vi "gyro -- async sweeper.vi"(11 "sweeper event pair":T4) -> ()   [LabVIEW 2018]
uses:
  publisher action.ctl
  data source action.ctl
  server talkback message type.ctl
  gyro -- async sweeper parameters.ctl
  freq scan type.ctl
  show-win- control.ctl
  server talkto message type.ctl
  server talk-to-back pair.ctl
panel:
  in  "Tab Control":enum32{"Page 1", "Page 2"}(tab)
  in  "sweeper parameters":T1={"delay-circle(msec)"=0, "N"=300, "scan type"=enum."linear", "gamma factor"=1.5, "history length"=1}
  in  "win":T3={"cen (Hz)"=32757.83435625395, "win (Hz)"=134.34356253945762, "left (Hz)"=32690.66257498422, "right (Hz)"=32825.00613752368}
  out "progress":i32(slide) min=0 max=300 step=1 scale=0.0..300.0
  out "stopped?":bool=TRUE
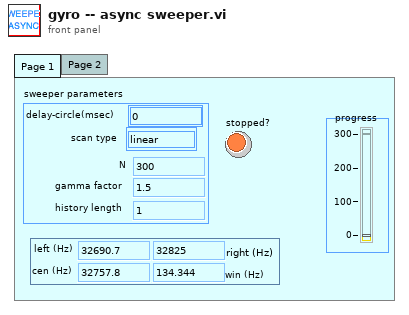
[diagram p1: front panel]
types:
  T1 = typedef "gyro -- async sweeper parameters.ctl" = cluster{"delay-circle(msec)":i64, "N":i64, "scan type":T2, "gamma factor":dbl, "history length":i64}
  T2 = typedef "freq scan type.ctl" = enum16{"linear", "arctan"}
  T3 = typedef "show-win- control.ctl" = cluster{"cen (Hz)":dbl, "win (Hz)":dbl, "left (Hz)":dbl, "right (Hz)":dbl}
  T4 = typedef "server talk-to-back pair.ctl" = cluster{"talkback event":refnum<user-event>, "talkto event":refnum<user-event>}
  T5 = typedef "publisher action.ctl" = enum16{"set", "get", "init", "check"}
  T6 = typedef "server talkback message type.ctl" = cluster{"message":enum16{"new", "void"}}
  T7 = typedef "data source action.ctl" = enum16{"set", "get", "init", "set-and-get", "init source"}
  T8 = enum16{"stop", "start", "update pars", "update request", "new", "launch", "exit", "get", "reset", "pause", "unpause"}
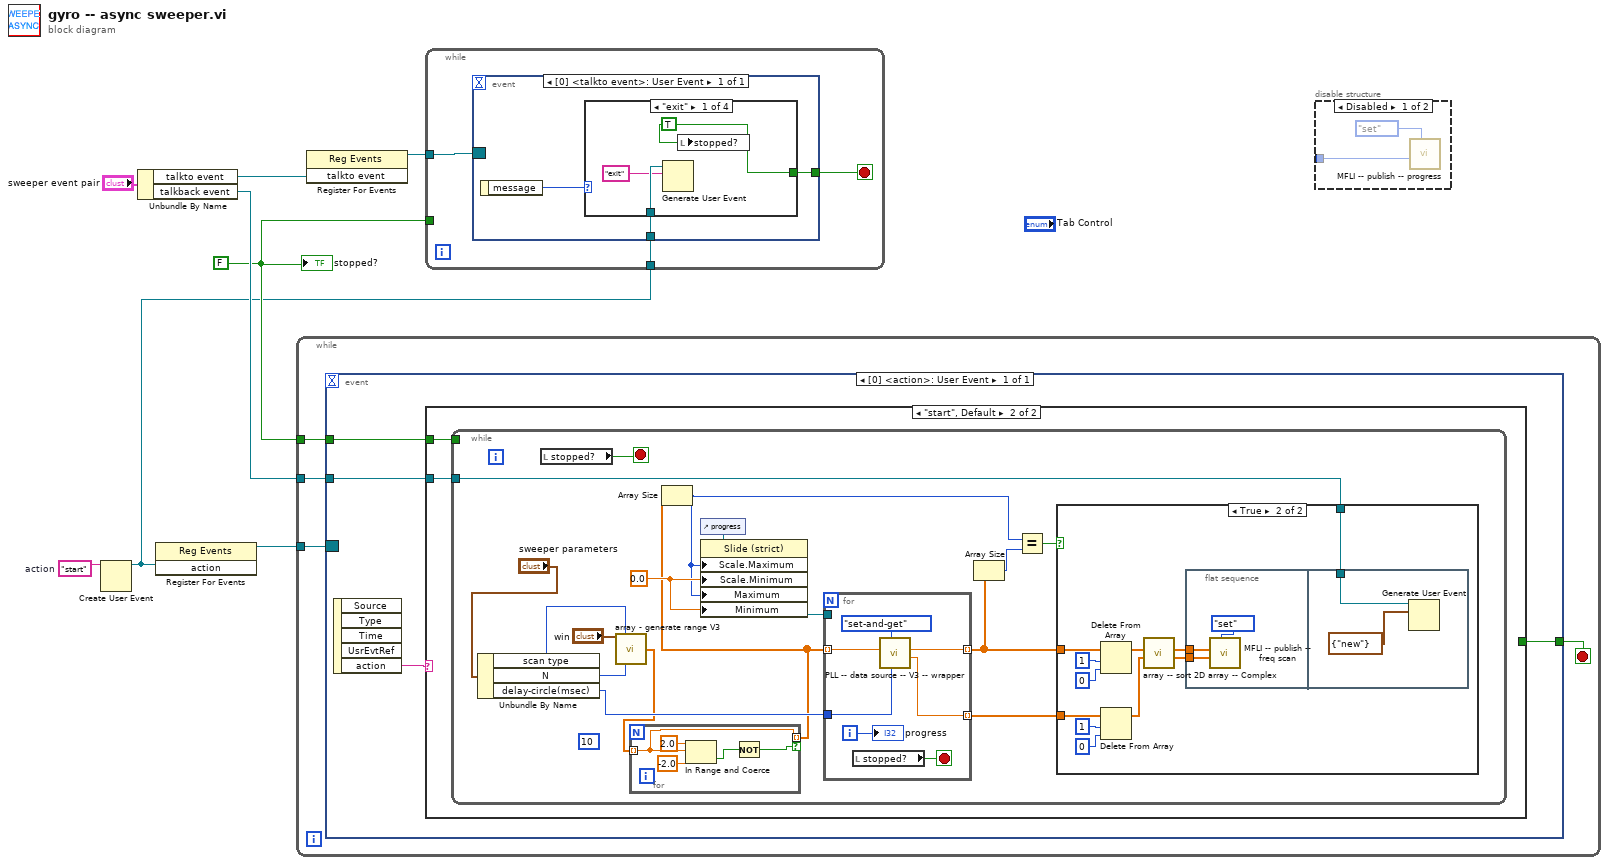
[diagram p0: block diagram]
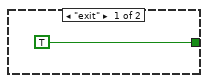
[diagram p2: hidden frame]
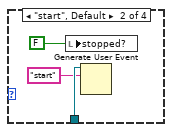
[diagram p5: hidden frame]
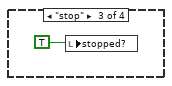
[diagram p6: hidden frame]
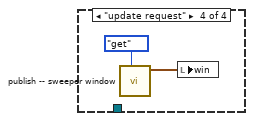
[diagram p7: hidden frame]
diagram:
  w3 = "start"  # action
  w2 = FALSE ("stop!")
  n1 = Create User Event(user event datatype=w3) -> (user event=w1:refnum<user-event>)  [unwired: 1 in, 1 out]
  n2 = Unbundle By Name("sweeper event pair") -> ("talkto event"=w6:refnum<user-event>, "talkback event"=w5:refnum<user-event>)
  n3 = register-events(w1) -> (reference out=w4:refnum<event-registration>)  [unwired: 2 in, 1 out]
  n4 = while {
    tunnel: w2 -> [w12]
    tunnel: w5 -> [w11]
    tunnel: w4 -> [w10]
    stop <- w9 stop-if-true
    n5 = event shown="[0] <action>: User Event" {
      selector: w10 -> [_]
      dyn-events: _ -> [_]
      timeout: _ -> [_]
      tunnel: w12 -> [w16]
      tunnel: w11 -> [w15]
      tunnel: [w13] -> w9
      event User Event {
        n6 = event-data() -> ("action"=w14:string)  [unwired: 1 in, 4 out]
        n7 = case shown="\"start\", Default" w14 {
          tunnel: w16 -> [_ w19]
          tunnel: w15 -> [_ w18]
          tunnel: [TRUE ("stop!") _] -> w13
          frame "exit" {
          }
          frame "start", Default {
            n8 = while {
              tunnel: w19 -> [_]
              tunnel: w18 -> [w34]
              stop <- w27 stop-if-true
              (unwired) 10 ("lower")
              w29 = 0.0 ("Scale.Range:Minimum")
              n9 = Unbundle By Name("sweeper parameters") -> ("scan type"=w33:T2, "N"=w22:i64, "delay-circle(msec)"=w32:i64)
              n10 = local read "stopped?"() -> (w27:bool)
              n11 = call "array - generate range V3.vi"("win"="win", "scan type"=w33, "N"=w22) -> ("Array"=w21:dbl[])  [unwired: 11 in, 1 out]
              n12 = for {
                tunnel: w21 -> [w39] mode=indexing
                tunnel: [w39] -> w20 mode=indexing if=w37
                n13 = In Range and Coerce(upper limit=2.0, x=w39, lower limit=-2.0) -> (In Range?=w38:bool)  [unwired: 1 out]
                n14 = Not(x=w38) -> (.not. x?=w37:bool)
              }
              n15 = Array Size(array=w20) -> (size(s)=w23:i32)
              n16 = control-ref of="progress"() -> (w31:refnum<vi>)
              n17 = property class="Slide (strict)"(reference=w31, "Scale.Maximum"=w23, "Scale.Minimum"=w29, "Maximum"=w23, "Minimum"=w29) -> (reference out=w30:refnum<vi>)  [unwired: 1 in, 1 out]
              n18 = for {
                tunnel: w20 -> [w60] mode=indexing
                tunnel: w32 -> [w62]
                tunnel: [w64] -> w36 mode=indexing
                tunnel: [w63] -> w26 mode=indexing
                tunnel: w30 -> [_]
                i -> [w59]
                stop <- w58 stop-if-true
                n19 = local read "stopped?"() -> (w58:bool)
                n20 = call "PLL -- data source -- V3 -- wrapper.vi"("set-get delay (msec)"=w62, "data source action"=data_source_action."set-and-get", "Freq in (Hz)"=w60) -> ("z out (V)"=w64:cdb, "Freq out (Hz)"=w63:dbl)  [unwired: 6 in, 1 out]
                "progress" <- w59
              }
              n21 = Array Size(array=w26) -> (size(s)=w24:i32)
              n22 = Equal?(x=w23, y=w24) -> (x = y?=w25:bool)
              n23 = case shown="True" w25 {
                tunnel: w36 -> [_ w48]
                tunnel: w26 -> [_ w47]
                tunnel: w34 -> [_ w42]
                frame False {
                }
                frame True {
                  n24 = Delete From Array(array=w47, length=1, index=0) -> (array with subset deleted=w46:dbl[])  [unwired: 1 out]
                  n25 = Delete From Array(array=w48, length=1, index=0) -> (array with subset deleted=w45:cdb[])  [unwired: 1 out]
                  n26 = call "array -- sort 2D array -- Complex.vi"("z In"=w45, "freq IN"=w46) -> ("z out"=w43:cdb[], "freq out"=w44:dbl[])  [unwired: 8 in]
                  n27 = flat-sequence {
                    tunnel: w43 -> [w54]
                    tunnel: w44 -> [w53]
                    tunnel: w42 -> [w57]
                    frame #0 {
                      n28 = call "MFLI -- publish -- freq scan.vi"("publisher action"=publisher_action."set", "Voltage IN (V)"=w54, "Freq IN (Hz)"=w53) -> ()  [unwired: 7 in, 2 out]
                    }
                    frame #1 {
                      n29 = Generate User Event(user event=w57, event data cluster=T6 {"message"=enum."new"} ("event data")) -> ()  [unwired: 2 in, 2 out]
                    }
                  }
                }
              }
            }
          }
        }
      }
    }
  }
  n30 = register-events(w6) -> (reference out=w8:refnum<event-registration>)  [unwired: 2 in, 1 out]
  n31 = while {
    tunnel: w8 -> [w67]
    tunnel: w2 -> [_]
    tunnel: w1 -> [w65]
    stop <- w66 stop-if-true
    n32 = event shown="[0] <talkto event>: User Event" {
      selector: w67 -> [_]
      dyn-events: _ -> [_]
      timeout: _ -> [_]
      tunnel: [w70] -> w66
      tunnel: w65 -> [w68]
      event User Event {
        n33 = event-data() -> ("message"=w69:T8)  [unwired: 1 in]
        n34 = case shown="\"exit\"" w69 {
          tunnel: [w73 _ _ _] -> w70
          tunnel: w68 -> [w72 w75 _ _]
          frame "exit" {
            w73 = TRUE ("stop!")
            n35 = Generate User Event(user event=w72, event data cluster="exit" ("event data")) -> ()  [unwired: 2 in, 2 out]
            n36 = local write "stopped?"(w73) -> ()
          }
          frame "start", Default {
            n37 = local write "stopped?"(FALSE ("stop!")) -> ()
            n38 = Generate User Event(user event=w75, event data cluster="start" ("event data")) -> ()  [unwired: 2 in, 2 out]
          }
          frame "stop" {
            n39 = local write "stopped?"(TRUE ("stop!")) -> ()
          }
          frame "update request" {
            n40 = call "publish -- sweeper window.vi"("publisher action"=publisher_action."get") -> ("win OUT"=w78:T3)  [unwired: 10 in]
            n41 = local write "win"(w78) -> ()
          }
        }
      }
    }
  }
  n42 = disable-structure shown="Disabled" {
    disable-tunnel: _ -> [w80 _]
    frame Disabled {
      n43 = call "MFLI -- publish -- progress.vi"("publisher action"=publisher_action."set", "num"=w80) -> ()  [unwired: 9 in, 1 out]
    }
    frame Enabled {
    }
  }
  "stopped?" <- w2
